vi "runPrefix.get.vi"(8 "error in (no error)":errorcluster, 11 "Run in":refnum<class "Run.lvclass">) -> (0 "error out":errorcluster, 2 "runPrefix":string, 3 "Run out":refnum<class "Run.lvclass">)   [LabVIEW 2020, in "Run.lvclass"]
uses:
  Run.lvclass
  Run.lvclass/Run.ctl
  a95c02fe-50a5-4945-b9d2-058883f2984e.vi
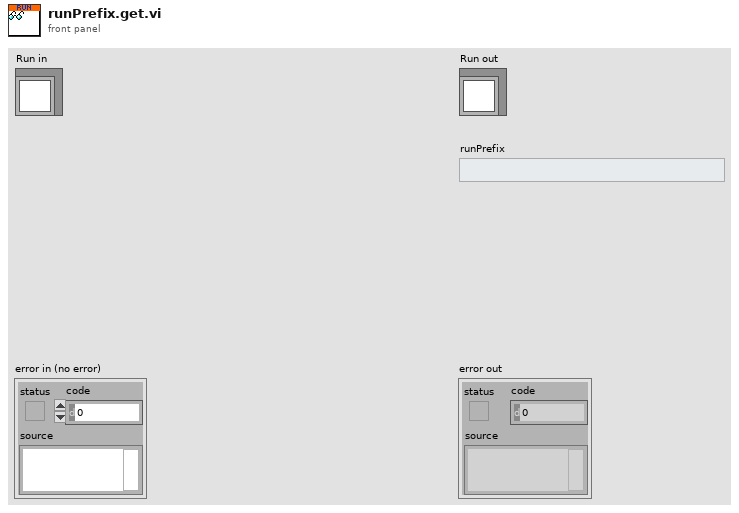
[diagram p1: front panel]
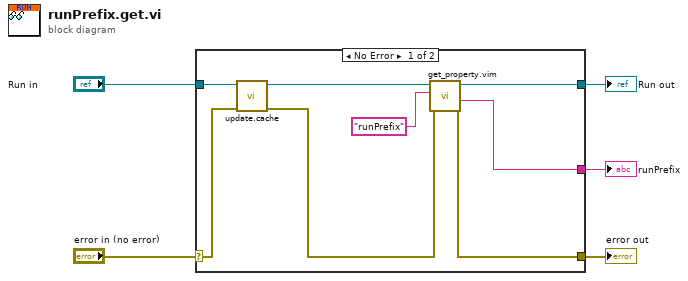
[diagram p0: block diagram]
diagram:
  n1 = case shown="No Error" "error in (no error)" {
    selector: "error in (no error)" -> [w13 w14]
    tunnel: [w7 w14] -> w4
    tunnel: [w9 w15] -> w2
    tunnel: "Run in" -> [w12 w15]
    tunnel: [w6 _] -> w1
    frame No Error {
      n2 = call "update.cache.vi"("error in"=w13, "Run in"=w12) -> ("error out"=w8:errorcluster, "Run out"=w10:refnum<class "Run.lvclass">)  [unwired: 8 in]
      n3 = call "get_property.vim"("error in"=w8, "Property Name"="runPrefix", "Run in"=w10) -> ("error out"=w7:errorcluster, "Value"=w6:string, "Run out"=w9:refnum<class "Run.lvclass">)  [unwired: 6 in]
    }
    frame Error {
    }
  }
  "error out" <- w4
  "Run out" <- w2
  "runPrefix" <- w1
